vi "Discover Plugins.vi"(6 "timeout (ms)":i32=5000, 8 "error in":errorcluster, 10 "update_metadata":bool, 11 "gRPC ID in":T4) -> (0 "error out":errorcluster, 2 "discovered_plugins":T1[](array[typedef]), 3 "gRPC ID out":T4)   [LabVIEW 2021, in "CIFPluginLoaderClientWrapper.lvlib"]
uses:
  CIFPluginLoaderClientWrapper.lvlib
  CIF_PluginLoader_client/CIF_PluginLoader_client.lvlib
  CIF_PluginLoader_client/RPC Messages/cif_pluginloader_DiscoverRequest.ctl
  <vilib>/gRPC/LabVIEW gRPC Library/Shared/grpcId.ctl
  <vilib>/gRPC/LabVIEW gRPC Library/grpc-lvsupport-release.lvlib
  CIF_PluginLoader_client/RPC Messages/cif_manager_PluginMetadata.ctl
  CIF_PluginLoader_client/RPC Messages/cif_common_Version.ctl
  CIF_PluginLoader_client/RPC Messages/cif_pluginloader_DiscoveredPlugin.ctl
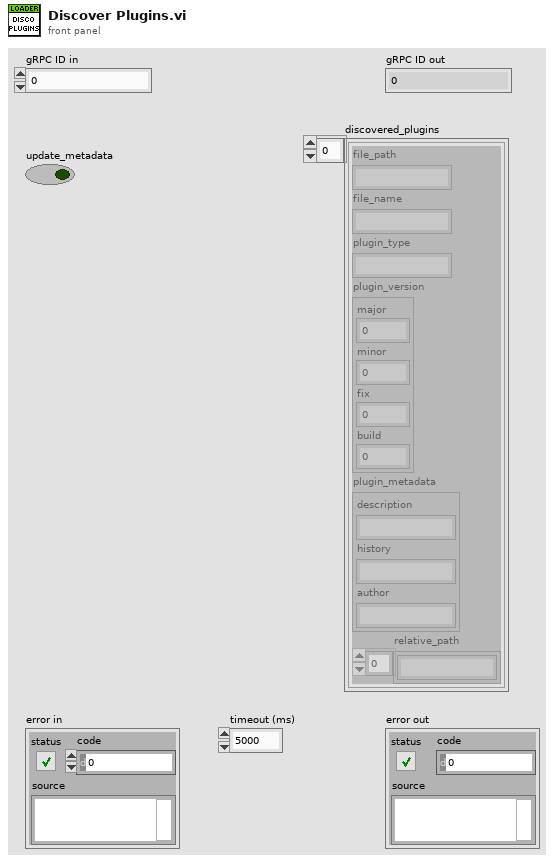
[diagram p1: front panel]
types:
  T1 = typedef "CIF_PluginLoader_client.lvlib/cif_pluginloader_DiscoveredPlugin.ctl" = cluster{"file_path":string, "file_name":string, "plugin_type":string, "plugin_version":T2, "plugin_metadata":T3, "relative_path":string[]}
  T2 = typedef "CIF_PluginLoader_client.lvlib/cif_common_Version.ctl" = cluster{"major":u32, "minor":u32, "fix":u32, "build":u32}
  T3 = typedef "CIF_PluginLoader_client.lvlib/cif_manager_PluginMetadata.ctl" = cluster{"description":string, "history":string, "author":string}
  T4 = typedef "grpc-lvsupport-release.lvlib/grpcId.ctl" = u64
  T5 = typedef "CIF_PluginLoader_client.lvlib/cif_pluginloader_DiscoverRequest.ctl" = cluster{"update_metadata":bool}
  T6 = typedef "CIF_PluginLoader_client.lvlib/cif_pluginloader_DiscoverResponse.ctl" = cluster{"discovered_plugins":T1[], "status":T7}
  T7 = typedef "CIF_PluginLoader_client.lvlib/cif_common_Status.ctl" = cluster{"code":i32, "message":string}
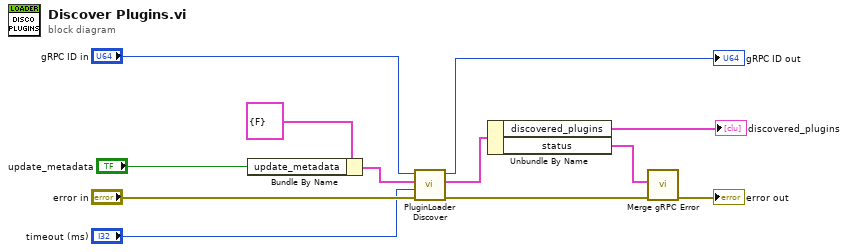
[diagram p0: block diagram]
diagram:
  n1 = Bundle By Name(cluster=T5 {"update_metadata"=FALSE} ("Request Data"), "update_metadata"="update_metadata") -> (w5:T5)
  n2 = call "PluginLoader Discover.vi"("error in"="error in", "timeout (ms)"="timeout (ms)", "Request Data"=w5, "gRPC ID"="gRPC ID in") -> ("error out"=w8:errorcluster, "Response Data"=w4:T6, "gRPC ID out"=→"gRPC ID out":T4)  [unwired: 5 in]
  n3 = Unbundle By Name(w4) -> ("discovered_plugins"=→"discovered_plugins":T1[], "status"=w3:T7)
  n4 = call "Merge gRPC Error.vi"("error in (no error)"=w8, "gRPC Error"=w3) -> ("error out"=→"error out":errorcluster)  [unwired: 9 in]
